vi "Example_BP Network_Curve Fitting.vi"() -> ()   [LabVIEW 2009]
uses:
  <vilib>/addons/Machine Learning/Supervised Learning/ml_BP_Terminal Condition.ctl
  <vilib>/Utility/miscctls.llb/LV3DPointTypeDef.ctl
  <vilib>/addons/Machine Learning/Visualization/Visualization (3D).vi
  <vilib>/addons/Machine Learning/Utilities/Training & Test Set (matrix-matrix).vi
  <vilib>/addons/Machine Learning/NILabs_MLT.lvlib
panel:
  in  "Stopping criteria":T1={"min MSE"=1e-05, "min delta MSE"=1e-08, "min step length"=1e-08, "max iteration"=5000.0}
  in  "# of hidden neurons":i32=10
  out "Data samples":refnum<vi>(3d-picture)
  out "mse":dbl
  # "Introduction:\nA Back-propagation (BP) neural network is applied to a 3-D surface fitting problem."
  # "(red: training samples; green: test samples)"
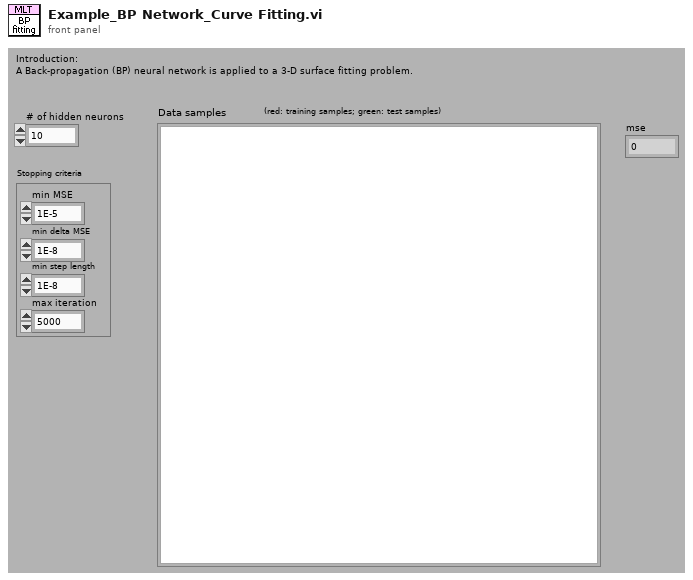
[diagram p1: front panel]
types:
  T1 = typedef "NILabs_MLT.lvlib/ml_BP_Terminal Condition.ctl" = cluster{"min MSE":dbl, "min delta MSE":dbl, "min step length":dbl, "max iteration":dbl}
  T2 = typedef "LV3DPointTypeDef.ctl" = cluster{"X":sgl, "Y":sgl, "Z":sgl}
  T3 = typedef "NILabs_MLT.lvlib/ml_BP_Project.ctl" = cluster{"Training Data":T4, "Normalize Info":T5, "3-layer NN":T6, "Ternimal Condition":T1}
  T4 = typedef "NILabs_MLT.lvlib/ml_BP_Data.ctl" = cluster{"dim in":i32, "dim out":i32, "# samples":i32, "Input":dbl[][], "Output":dbl[][]}
  T5 = typedef "NILabs_MLT.lvlib/ml_BP_Normalize Data.ctl" = cluster{"input min":dbl[], "input max":dbl[], "output min":dbl[], "output max":dbl[]}
  T6 = typedef "NILabs_MLT.lvlib/ml_BP_3layer Feedforward.ctl" = cluster{"# input neuron ":i32, "# hidden neuron":i32, "# output neuron":i32, "Weight (I->H)":dbl[][], "Weight (H->O)":dbl[][], "Output":dbl[][], "Hidden Out":dbl[][], "Derivation Output":dbl[][], "Derivation Hidden":dbl[][], "dw (I->H)":dbl[][], "dw (H->O)":dbl[][]}
  T7 = typedef "NI_Matrix.lvlib/RealMatrix.ctl" = dbl[][]
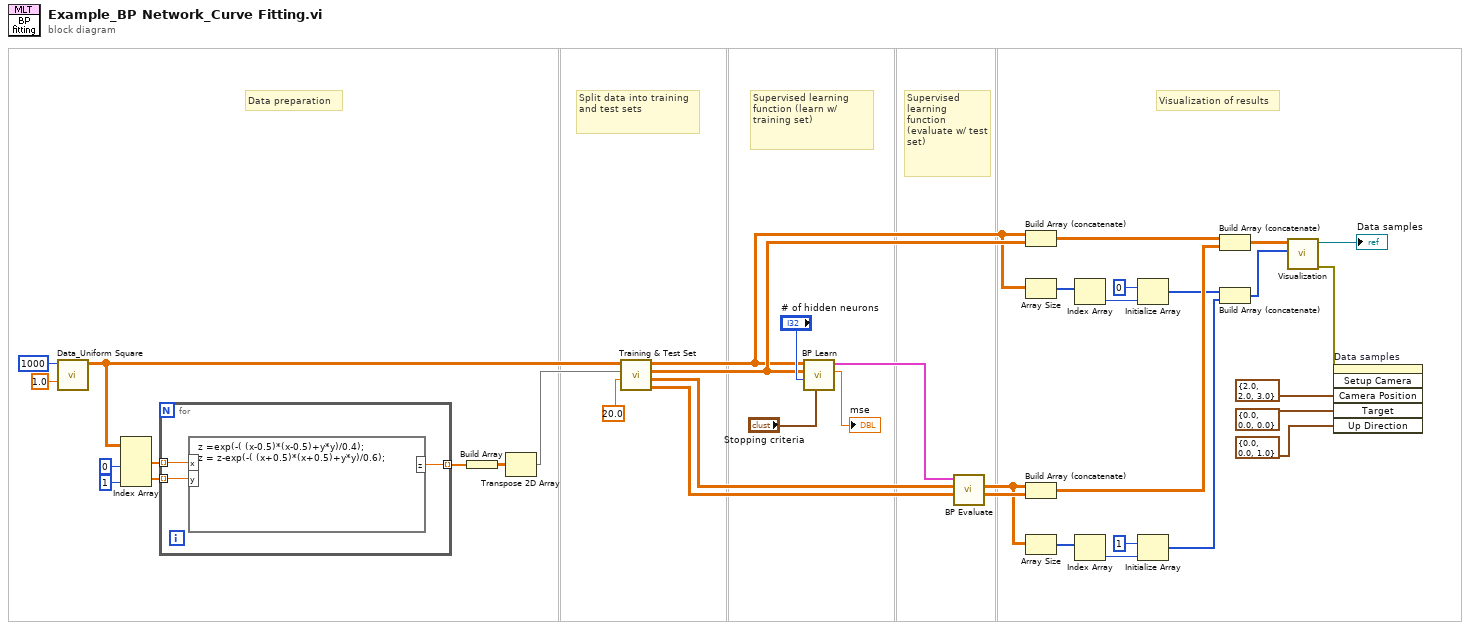
[diagram p0: block diagram]
diagram:
  # "Visualization of results"
  # "Supervised learning function (evaluate w/ test set)"
  # "Supervised learning function (learn w/ training set)"
  # "Split data into training and test sets"
  # "Data preparation"
  n1 = call "Data_Uniform Square.vi"("amplitude"=1.0, "# of points"=1000) -> ("Data"=w38:dbl[][])  [unwired: 8 in, 1 out]
  n2 = Index Array(array=w38, index (col) #1=0 ("disabled index (col)"), index (col) #2=1 ("index (col)")) -> (element #1=w35:dbl[], element #2=w34:dbl[])  [unwired: 2 in]
  n3 = for {
    tunnel: w35 -> [w41] mode=indexing
    tunnel: w34 -> [w40] mode=indexing
    tunnel: [w39] -> w33 mode=indexing
    n4 = formula code="z =exp(-( (x-0.5)*(x-0.5)+y*y)/0.4);\nz = z-exp(-( (x+0.5)*(x+0.5)+y*y)/0.6);"("x"=w41, "y"=w40) -> ("z"=w39:dbl)
  }
  n5 = Build Array(w33) -> (w32:dbl[][])
  n6 = Transpose 2D Array(2D array=w32) -> (transposed array=w31:dbl[][])
  n7 = call-poly <vilib>:"Training & Test Set.vi"("percent"=20.0, "Samples out"=w31, "Samples in"=w38) -> ("Test Set Out"=w25:dbl[][], "Test Set In"=w26:dbl[][], "Training Set Out"=w24:dbl[][], "Training Set In"=w19:dbl[][])  [unwired: 5 in]
  n8 = call <vilib>:"BP Learn.vi"("Stopping Criteria"="Stopping criteria", "# of hidden neuron"="# of hidden neurons", "Training outputs"=w24, "Training data samples"=w19) -> ("mse"=→"mse":dbl, "BP Project"=w27:T3)  [unwired: 4 in, 2 out]
  n9 = call <vilib>:"BP Evaluate.vi"("Test outputs"=w25, "Test data samples"=w26, "BP Project"=w27) -> ("NN outputs"=w23:dbl[][], "Test data samples dup"=w18:dbl[][])  [unwired: 4 in, 3 out]
  n10 = Build Array (concatenate)(w19, w24) -> (w22:T7)
  n11 = Array Size(array=w19) -> (size(s)=w17:i32[])
  n12 = Build Array (concatenate)(w18, w23) -> (w21:T7)
  n13 = Array Size(array=w18) -> (size(s)=w16:i32[])
  n14 = Index Array(array=w17) -> (element=w15:i32)  [unwired: 1 in]
  n15 = Index Array(array=w16) -> (element=w12:i32)  [unwired: 1 in]
  n16 = Initialize Array(0 ("element"), w15) -> (w11:i32[])
  n17 = Initialize Array(1 ("element"), w12) -> (w10:i32[])
  n18 = Build Array (concatenate)(w22, w21) -> (w20:T7)
  n19 = Build Array (concatenate)(w11, w10) -> (w9:i32[])
  n20 = call-poly <vilib>:"Visualization.vi"("Class labels"=w9, "Data samples"=w20) -> ("error out"=w4:errorcluster, "3D Picture"=→"Data samples":refnum<vi>)  [unwired: 8 in]
  n21 = invoke on="Data samples" class="SceneGraphDisp (strict)" method="Setup Camera"(error in=w4, "Camera Position"=T2 {"X"=2.0, "Y"=2.0, "Z"=3.0}, "Target"=T2 {"X"=0.0, "Y"=0.0, "Z"=0.0} ("Camera Position"), "Up Direction"=T2 {"X"=0.0, "Y"=0.0, "Z"=1.0} ("Camera Position")) -> ()  [unwired: 2 in, 6 out]
